vi "dfd_FXP Lattice Allpass (basic) with IS.vi"(6 "state in":i64[](array[numeric]), 7 "FXPOPs":T5[](array[typedef]) {"source" items=["Coef a/k"=0, "Coef b/v"=7, "Input"=1, "Output"=2, "Multiplicand"=3, "Product"=4, "Sum"=5, "Delay"=6, "Gain"=8]}, 8 "filtering statistics in":T4(array[cluster]) {"statistics information"."min value" format="%.2f"; "statistics information"."max value" format="%.2f"; "Quantizer Source" items=["Coefficients a/k"=0, "Coefficients b/v"=7, "Input"=1, "Output"=2, "Multiplicand"=3, "Product"=4, "Sum"=5, "Delay"=6]}, 10 "coef k":T7, 11 "X":T7) -> (0 "filtering statistics out":T4(array[cluster]) {"statistics information"."min value" format="%.2f"; "statistics information"."max value" format="%.2f"; "Quantizer Source" items=["Coefficients a/k"=0, "Coefficients b/v"=7, "Input"=1, "Output"=2, "Multiplicand"=3, "Product"=4, "Sum"=5, "Delay"=6]}, 3 "filtered X":T7, 4 "state out":i64[](array[numeric]))   [LabVIEW 2017, in "NI_DigFilter_FXP.lvlib"]
uses:
  <vilib>/addons/Digital Filter Design/NI_DigFilter_FXP.lvlib
  <vilib>/addons/Digital Filter Design/_Objects.llb/dfd_DFXP Data Type (vector).ctl
  <vilib>/addons/Digital Filter Design/_Objects.llb/dfd_DFXP Operation Parameter.ctl
  <vilib>/addons/Digital Filter Design/_Objects.llb/dfd_Internal Quantization Srcs.ctl
  <vilib>/addons/Digital Filter Design/_Objects.llb/DFD Quantization Sources.ctl
  <vilib>/addons/Digital Filter Design/_Objects.llb/DFD FXP Statistics Data.ctl
  <vilib>/addons/Digital Filter Design/_Objects.llb/dfd_DFXP Data Type (scaler).ctl
  <vilib>/addons/Digital Filter Design/NI_DigFilterLicensed.lvlib
panel:
  in  "DFXP Value":T1={"value"=0, "wl"=0, "iwl"=0, "Signed"=TRUE} {"value" format="%.0x"}
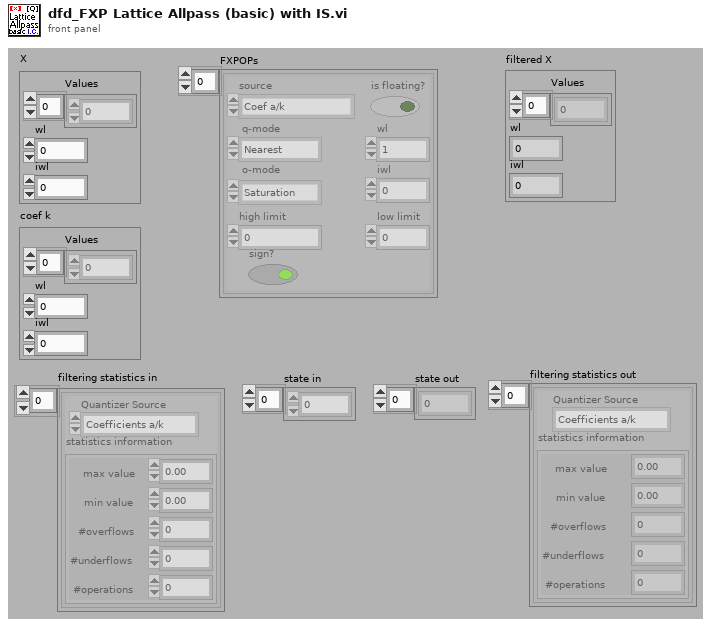
[diagram p1: front panel]
types:
  T1 = typedef "dfd_DFXP Data Type (scaler).ctl" = cluster{"value":i64, "wl":i16, "iwl":i16, "Signed":bool}
  T2 = typedef "NI_DigFilterLicensed.lvlib/DFD Quantization Sources.ctl" = u16
  T3 = typedef "NI_DigFilterLicensed.lvlib/DFD FXP Statistics Data.ctl" = cluster{"max value":ext, "min value":ext, "#overflows":i32, "#underflows":i32, "#operations":i32}
  T4 = cluster{"Quantizer Source":T2, "statistics information":T3}[]
  T5 = typedef "dfd_DFXP Operation Parameter.ctl" = cluster{"source":T6, "is floating?":bool, "o-mode":enum16{"Saturation", "Wrap"}, "q-mode":enum16{"Nearest", "Truncation"}, "wl":i16, "high limit":i64, "low limit":i64, "iwl":i16, "sign?":bool}
  T6 = typedef "NI_DigFilterLicensed.lvlib/dfd_Internal Quantization Srcs.ctl" = u16
  T7 = typedef "dfd_DFXP Data Type (vector).ctl" = cluster{"Values":i64[], "wl":i16, "iwl":i16}
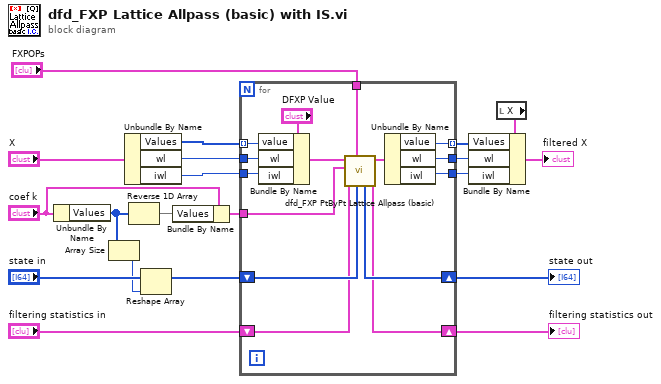
[diagram p0: block diagram]
diagram:
  n1 = Unbundle By Name("coef k") -> ("Values"=w10:i64[])
  n2 = Array Size(array=w10) -> (size(s)=w15:i32)
  n3 = Unbundle By Name("X") -> ("Values"=w7:i64[], "wl"=w6:i16, "iwl"=w5:i16)
  n4 = Reverse 1D Array(array=w10) -> (reversed array=w16:i64[])
  n5 = Reshape Array("state in", w15) -> (w19:i64[])
  n6 = Bundle By Name(cluster="coef k", "Values"=w16) -> (w9:T7)
  n7 = for {
    tunnel: w7 -> [w35] mode=indexing
    tunnel: w9 -> [w33]
    shift-right: [w31] -> w17
    shift-left: w19 -> [w32]
    tunnel: "FXPOPs" -> [w34]
    tunnel: [w23] -> w13 mode=indexing
    shift-right: [w28] -> w11
    shift-left: "filtering statistics in" -> [w29]
    tunnel: w6 -> [w25]
    tunnel: w5 -> [w24]
    tunnel: [w22] -> w2
    tunnel: [w21] -> w1
    n8 = Bundle By Name(cluster="DFXP Value", "value"=w35, "wl"=w25, "iwl"=w24) -> (w27:T1)
    n9 = call <vilib>:"dfd_FXP PtByPt Lattice Allpass (basic).vi"("state in"=w32, "FXPOPs"=w34, "filtering statistics in"=w29, "coef k[M..1]"=w33, "x"=w27) -> ("filtering statistics out"=w28:T4, "filtered x"=w30:T1, "state out"=w31:i64[])  [unwired: 4 out]
    n10 = Unbundle By Name(w30) -> ("value"=w23:i64, "wl"=w22:i16, "iwl"=w21:i16)
  }
  "state out" <- w17
  "filtering statistics out" <- w11
  n11 = local read "X"() -> (w3:T7)
  n12 = Bundle By Name(cluster=w3, "Values"=w13, "wl"=w2, "iwl"=w1) -> (→"filtered X":T7)
